vi "GetMotorInfoProperties.vi"(8 "error in (no error)":errorcluster, 10 "Channel Properties":T1[](array[typedef])) -> (0 "error out":errorcluster, 3 "Selected Channel Properties":T1[](array[typedef]))   [LabVIEW 2017, in "McsaAnalysisFunctions.lvlib"]
uses:
  <vilib>/addons/InsightCM/MessageBus/Base/controls/KeyValuePair.ctl
  <vilib>/addons/InsightCM/Utilities/Analysis/MCSA/McsaAnalysisFunctions.lvlib
  <vilib>/addons/InsightCM/Utilities/PropertyHelpers/PropertyHelpers.lvlib
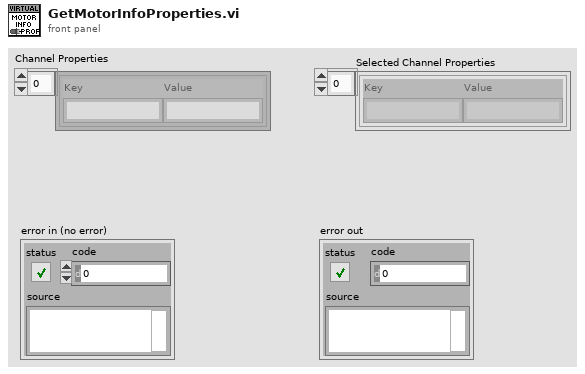
[diagram p1: front panel]
types:
  T1 = typedef "KeyValuePair.ctl" = cluster{"Key":string, "Value":string}
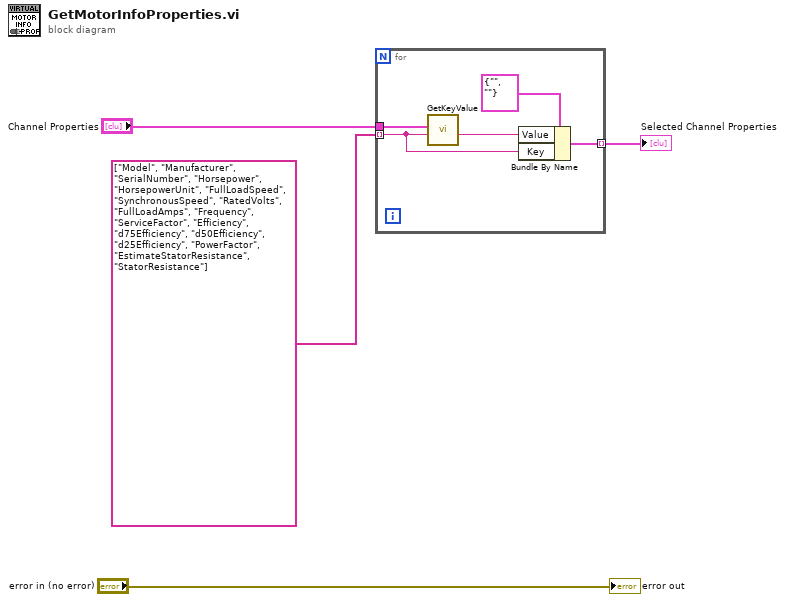
[diagram p0: block diagram]
diagram:
  n1 = for {
    tunnel: "Channel Properties" -> [w9]
    tunnel: string[] ["Model", "Manufacturer", "SerialNumber", "Horsepower", "HorsepowerUnit", "FullLoadSpeed", "SynchronousSpeed", "RatedVolts", "FullLoadAmps", "Frequency", "ServiceFactor", "Efficiency", "d75Efficiency", "d50Efficiency", "d25Efficiency", "PowerFactor", "EstimateStatorResistance", "StatorResistance"] -> [w6] mode=indexing
    tunnel: [w5] -> w1 mode=indexing
    n2 = call <vilib>:"GetKeyValue.vi"("key"=w6, "key value pairs"=w9) -> ("value"=w7:string)  [unwired: 7 in, 2 out]
    n3 = Bundle By Name(cluster=T1 {"Key"="", "Value"=""}, "Value"=w7, "Key"=w6) -> (w5:T1)
  }
  "Selected Channel Properties" <- w1
  "error out" <- "error in (no error)"
